vi "Generate SendInput Data.vi"(8 "error in (no error)":errorcluster, 11 "Array":u16[](array[numeric])) -> (0 "Error Out":errorcluster, 3 "Key Press Array":u8[][](array[numeric]))   [LabVIEW 2020, in "MacroAssert.lvlib" / "Win Util.lvlib"]
uses:
  Win Util.lvlib
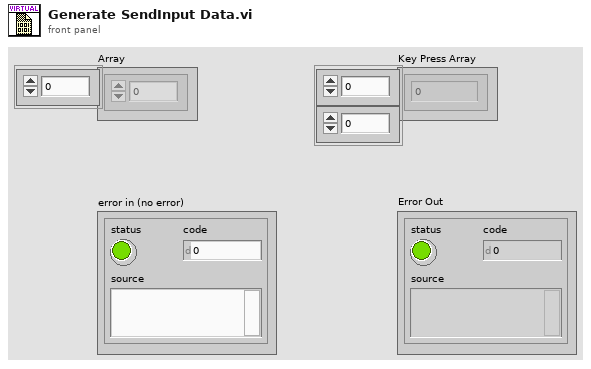
[diagram p1: front panel]
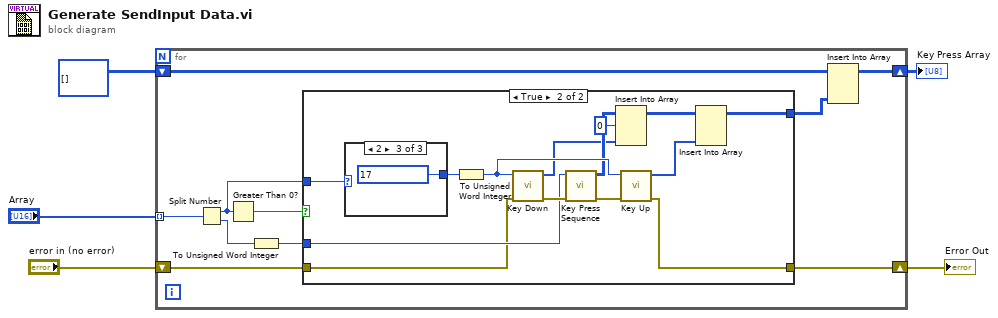
[diagram p0: block diagram]
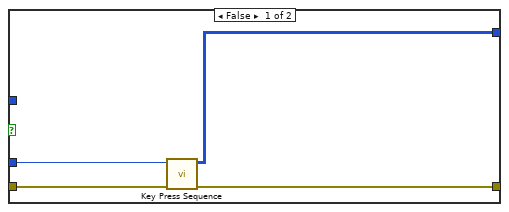
[diagram p2: hidden frame]
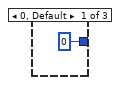
[diagram p3: hidden frame]
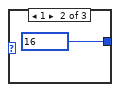
[diagram p4: hidden frame]
diagram:
  n1 = for {
    tunnel: "Array" -> [w15] mode=indexing
    shift-right: [w8] -> w3
    shift-left: u8[][] [] ("Key Press Array") -> [w9]
    shift-right: [w6] -> w1
    shift-left: "error in (no error)" -> [w7]
    n2 = Split Number(x=w15) -> (hi(x)=w13:u8, lo(x)=w12:u8)
    n3 = Greater Than 0?(x=w13) -> (x > 0?=w14:bool)
    n4 = To Unsigned Word Integer(number=w12) -> (unsigned 16bit integer=w11:u16)
    n5 = case shown="True" w14 {
      tunnel: w13 -> [_ w33]
      tunnel: w11 -> [w19 w31]
      tunnel: [w18 w23] -> w10
      tunnel: w7 -> [w17 w22]
      tunnel: [w16 w21] -> w6
      frame False {
        n6 = call "Key Press Sequence.vi"("Error In"=w17, "Vk"=w19) -> ("error out"=w16:errorcluster, "Key Press Array"=w18:u8[][])  [unwired: 8 in]
      }
      frame True {
        n7 = case shown="2" w33 {
          tunnel: [u8 0 ("Key") u8 16 ("Key") u8 17 ("Key")] -> w29
          frame 0, Default {
          }
          frame 1 {
          }
          frame 2 {
          }
        }
        n8 = To Unsigned Word Integer(number=w29) -> (unsigned 16bit integer=w28:u16)
        n9 = call "Key Down.vi"("error in (no error)"=w22, "Vk"=w28) -> ("error out"=w32:errorcluster, "INPUT"=w26:u8[])  [unwired: 8 in]
        n10 = call "Key Press Sequence.vi"("Error In"=w32, "Vk"=w31) -> ("error out"=w30:errorcluster, "Key Press Array"=w27:u8[][])  [unwired: 8 in]
        n11 = Insert Into Array(array=w27, index (row)=0, new element=w26) -> (w25:u8[][])  [unwired: 1 in]
        n12 = call "Key Up.vi"("error in (no error)"=w30, "Vk"=w28) -> ("error out"=w21:errorcluster, "INPUT"=w24:u8[])  [unwired: 8 in]
        n13 = Insert Into Array(array=w25, new element=w24) -> (w23:u8[][])  [unwired: 2 in]
      }
    }
    n14 = Insert Into Array(array=w9, new element=w10) -> (w8:u8[][])  [unwired: 2 in]
  }
  "Error Out" <- w1
  "Key Press Array" <- w3
